vi "Dio64DeviceNumber.vi"(11 "Action":enum16{"increment", "deincrement"}(ring)) -> (2 "Numeric":i32)   [LabVIEW 2009, in "Hardware.lvlib" / "Channels.lvlib"]
uses:
  Channels.lvlib
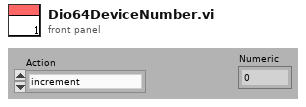
[diagram p1: front panel]
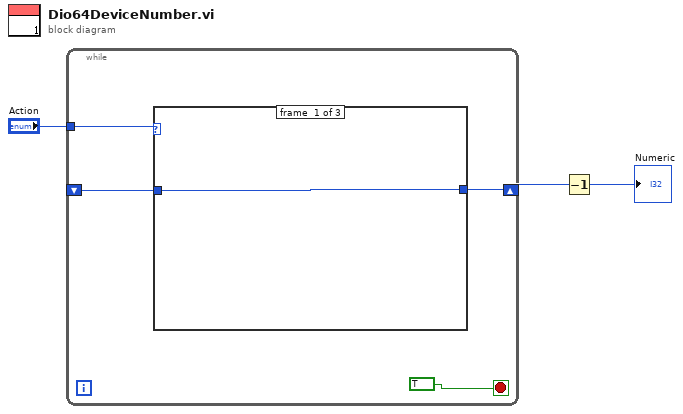
[diagram p0: block diagram]
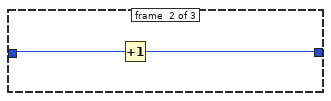
[diagram p2: hidden frame]
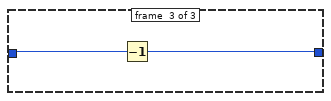
[diagram p3: hidden frame]
diagram:
  n1 = while {
    tunnel: "Action" -> [w7]
    shift-right: [w5] -> w2
    shift-left: _ -> [w4]
    stop <- TRUE stop-if-true
    n2 = case shown="\"deincrement\"" w7 {
      tunnel: [w8 w9 w11] -> w5
      tunnel: w4 -> [w8 w10 w12]
      frame #0 {
      }
      frame #1 {
        n3 = Increment(x=w10) -> (x+1=w9:i32)
      }
      frame #2 {
        n4 = Decrement(x=w12) -> (x-1=w11:i32)
      }
    }
  }
  n5 = Decrement(x=w2) -> (x-1=→"Numeric":i32)
